vi "freq PID point derivative.vi"(0 "Upper limit":fxp<+/-,26,10>, 1 "Lower limit":fxp<+/-,26,10>, 4 "final filter coeff":i32[](array[numeric])=[-955995012, 2025731616, 1001305, -1023351008, 2092954700, 1034533], 6 "DC offset":i16, 7 "Input":i16, 8 "Reset Integral":bool, 9 "P gain":fxp<+/-,32,11>, 10 "I gain":fxp<+/-,32,11>, 11 "D gain":fxp<+/-,32,11>) -> (2 "PID Output":fxp<+/-,26,10> format="%.26g")   [LabVIEW 2020]
uses:
  <vilib>/rvi/FXPMathLib/basic elements/FxpIntAccumulator/subVIs/nifxpmath_IntAccumulator_SimConfig.ctl
  <vilib>/rvi/FXPMathLib/basic elements/FxpIntAccumulator/simVIs/DllFxpIntAccumulator_sub.vi
  <vilib>/rvi/FXPMathLib/basic elements/FxpIntAccumulator/XNode/nifxpmath_IntAccumulator.xnode
  <vilib>/rvi/Analysis/measure/butterworth/XNode/niFpgaButterworthFilter.xnode
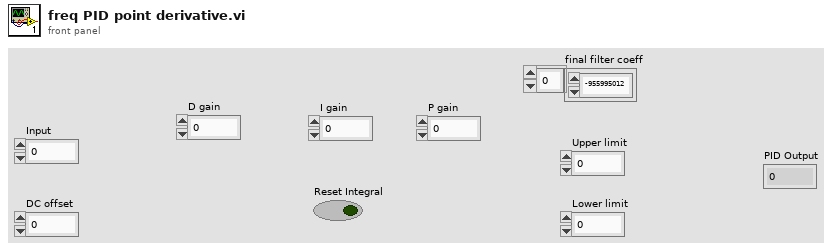
[diagram p1: front panel]
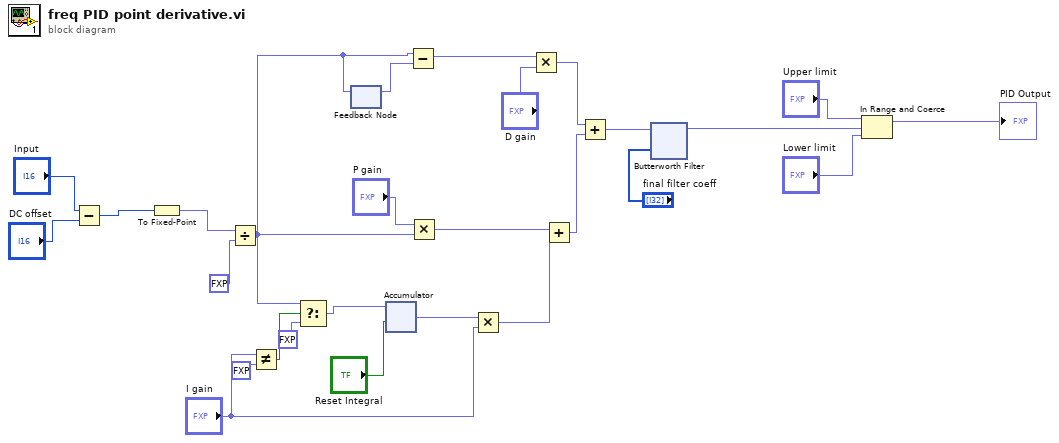
[diagram p0: block diagram]
diagram:
  n1 = Subtract(x="Input", y="DC offset") -> (x-y=w8:i16)
  n2 = To Fixed-Point(number=w8) -> (fixed-point=w9:fxp<+/-,32,16>)  [unwired: 1 in]
  n3 = Divide(x=w9, y=fxp<+,1,7> 64.0) -> (x/y=w1:fxp<+/-,26,10>)
  n4 = Not Equal?(x="I gain", y=fxp<+/-,16,16> 0.0) -> (x != y?=w18:bool)
  n5 = Select(t=w1, s=w18, f=fxp<+/-,26,10> 0.0) -> (s? t:f=w16:fxp<+/-,26,10>)
  n6 = feedback #1() -> (w2:fxp<+/-,26,10>)  [unwired: 1 in]
  n7 = feedback-in #1(w1) -> ()
  n8 = xnode "Accumulator"("x"=w16, "load (F)"="Reset Integral") -> ("s"=w27:fxp<+/-,33,17>)  [unwired: 3 in, 1 out]
  n9 = Subtract(x=w1, y=w2) -> (x-y=w3:fxp<+/-,27,11>)
  n10 = Multiply(x="P gain", y=w1) -> (x*y=w15:fxp<+/-,26,10>)
  n11 = Multiply(x=w27, y="I gain") -> (x*y=w24:fxp<+/-,26,10>)
  n12 = Multiply(x=w3, y="D gain") -> (x*y=w14:fxp<+/-,26,10>)
  n13 = Add(x=w15, y=w24) -> (x+y=w23:fxp<+/-,26,10>)
  n14 = Add(x=w14, y=w23) -> (x+y=w11:fxp<+/-,26,10>)
  n15 = xnode "Butterworth Filter"("input data"=w11, "scaled coefficients"="final filter coeff") -> ("output data"=w7:fxp<+/-,26,10>)  [unwired: 1 in]
  n16 = In Range and Coerce(upper limit="Upper limit", x=w7, lower limit="Lower limit") -> (coerced(x)=→"PID Output":fxp<+/-,26,10>)  [unwired: 1 out]
